vi "例6-6.vi"() -> ()   [LabVIEW 2019]
uses:
  <vilib>/measure/mascope.llb/Cycle Average and RMS 1 chan.vi
  <vilib>/measure/NI_MABase.lvlib
  <vilib>/measure/NI_MAPro.lvlib
panel:
  in  "停止":bool
  out "波形图":waveform(dbl)(graph)
  out "周期均方根":sgl format="%04_3g"
  out "周期平均值":sgl format="%04_1f"
  in  "采样点数":dbl=1000.0
  in  "采样频率":dbl=1000.0
  in  "信号频率":dbl=5.0
  in  "信号幅值":dbl=1.0
  # "输入参数"
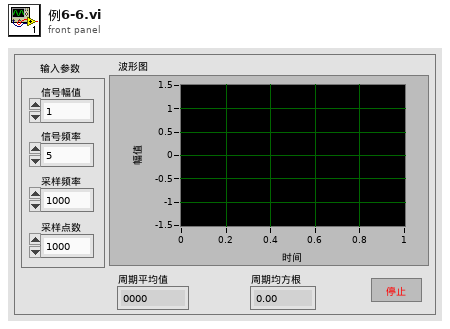
[diagram p1: front panel]
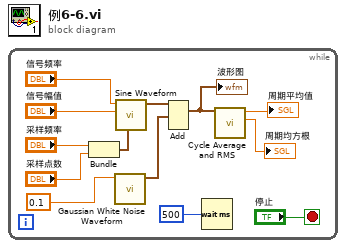
[diagram p0: block diagram]
diagram:
  n1 = while {
    stop <- "停止" stop-if-true
    n2 = Bundle("采样频率"="采样频率", "采样点数"="采样点数") -> (w8:cluster{"采样频率":dbl, "采样点数":dbl})  [unwired: 1 in]
    n3 = call <vilib>:"Gaussian White Noise Waveform.vi"("standard deviation"=0.1) -> ("signal out"=w5:waveform(dbl))  [unwired: 9 in, 1 out]
    n4 = call <vilib>:"Sine Waveform.vi"("sampling info"=w8, "amplitude"="信号幅值", "frequency"="信号频率") -> ("signal out"=w6:waveform(dbl))  [unwired: 7 in, 1 out]
    n5 = Add(1:w5, 2:w6) -> (0:w4:waveform(dbl))  [unwired: 1 in, 1 out]
    "波形图" <- w4
    n6 = Wait (ms)(milliseconds to wait=500) -> ()  [unwired: 1 out]
    n7 = call-poly <vilib>:"Cycle Average and RMS.vi"("signal in"=w4) -> ("cycle RMS"=→"周期均方根":dbl, "cycle average"=→"周期平均值":dbl)  [unwired: 7 in, 2 out]
  }
